vi "Peg-in-hole 2015-03-10 data.vi"() -> ()   [LabVIEW 2013]
uses:
  <vilib>/Analysis/baseanly.llb/Mean (DBL).vi
  <vilib>/Analysis/NI_AALBase.lvlib
  <vilib>/Analysis/NI_AALPro.lvlib
  <vilib>/gmath/NI_Gmath.lvlib
panel:
  in  "Times":dbl[](array[numeric])=[45.5, 55.1, 25.05, 25.0, 25.152, 25.451, 25.3, 25.35, 25.1, 25.25, 14.55, 25.45, 34.85, 25.55, 14.8, 25.15, 86.1, 25.55, 15.2, 25.5, 25.2, 25.201, 15.05, 25.45, 15.0, 25.8, 15.05, 25.1, 15.1, 25.85, 14.9, 25.7, 25.05, 25.1, 46.0, 25.9, 15.3, 25.45, 25.2, 25.601, 14.9, 24.95, 15.2, 25.0, 45.95, 25.25, 385.0, 25.65, 15.3, 25.4, 15.2, 25.7, 14.8, 25.1, 46.75, 25.85, 15.35, 25.1, 15.35, 25.95, 15.6, 25.55, 15.45, 25.45, 14.9, 14.9, 15.1, 15.35, 14.8, 15.05, 56.95, 25.7, 15.0, 15.15, 14.95, 25.899, 15.0, 25.15, 15.4, 15.251, 14.95, 25.6, 15.4, 15.5, 15.15, 14.95, 15.15, 15.25, 15.3, 15.35, 15.251, 15.8, 15.0, 15.05, 15.25, 15.55, 15.55, 15.65, 15.051, 15.5, 15.0, 15.0, 15.1, 15.45, 15.1, 15.15, 15.05, 25.15, 15.15, 15.25, 15.25, 15.1, 14.9, 15.25, 14.85, 15.35, 14.95, 25.85, 15.3, 15.8, 15.2, 15.2, 14.9, 15.3, 14.85, 15.55, 15.25, 15.35, 15.25, 15.3, 14.9, 15.3, 14.85, 15.45, 14.85, 15.3, 15.1, 15.3, 15.05, 15.851]
  in  "y":dbl
  out "correlation coefficient r":dbl
  out "offset":dbl
  out "power":dbl
  out "amplitude":dbl
  out "XY Graph":cluster{cluster{dbl, "mean":dbl}[]}[](graph)
  # "Data using two taught points\n& intervening joint pose"
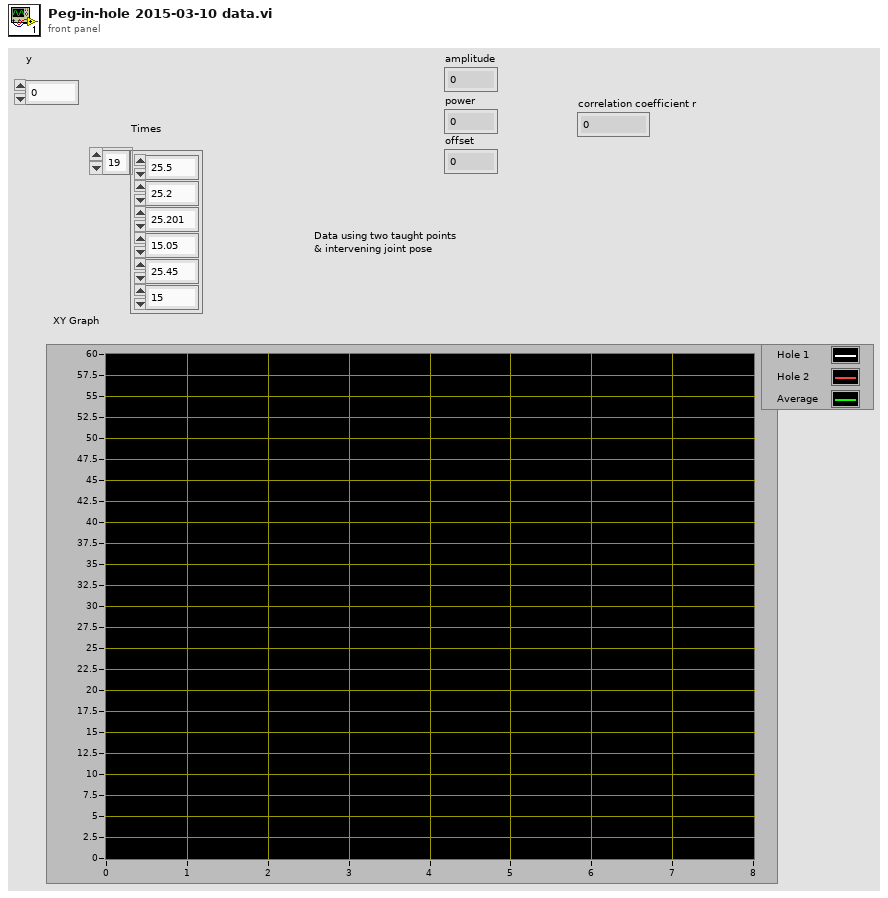
[diagram p1: front panel]
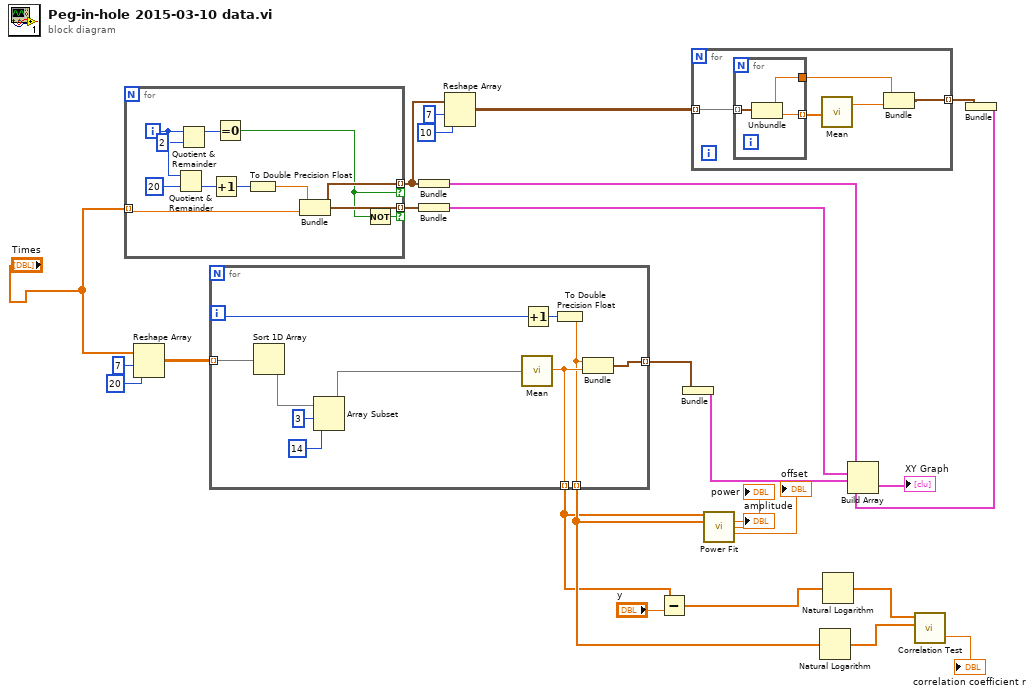
[diagram p0: block diagram]
diagram:
  n1 = for {
    tunnel: "Times" -> [w27] mode=indexing
    tunnel: [w30] -> w22 mode=indexing if=w28
    tunnel: [w30] -> w5 mode=indexing if=w29
    i -> [w33]
    n2 = Quotient & Remainder(x=w33, y=20) -> (floor(x/y)=w36:i32)  [unwired: 1 out]
    n3 = Quotient & Remainder(x=w33, y=2) -> (x-y*floor(x/y)=w31:i32)  [unwired: 1 out]
    n4 = Increment(x=w36) -> (x+1=w35:i32)
    n5 = Equal To 0?(x=w31) -> (x = 0?=w29:bool)
    n6 = To Double Precision Float(number=w35) -> (double precision float=w34:dbl)
    n7 = Bundle(w34, w27) -> (w30:cluster{dbl, dbl})  [unwired: 1 in]
    n8 = Not(x=w29) -> (.not. x?=w28:bool)
  }
  n9 = Reshape Array("Times", 7 ("dimension size"), 20 ("dimension size")) -> (w24:dbl[][])
  n10 = for {
    tunnel: w24 -> [w42] mode=indexing
    tunnel: [w45] -> w23 mode=indexing
    tunnel: [w44] -> w10 mode=indexing
    tunnel: [w43] -> w14 mode=indexing
    i -> [w47]
    n11 = Sort 1D Array(array=w42) -> (sorted array=w39:dbl[])
    n12 = Array Subset(array=w39, index=3, length=14) -> (w38:dbl[])
    n13 = call-poly <vilib>:"Mean.vi"("X"=w38) -> ("mean"=w44:dbl)  [unwired: 1 out]
    n14 = Increment(x=w47) -> (x+1=w46:i32)
    n15 = To Double Precision Float(number=w46) -> (double precision float=w43:dbl)
    n16 = Bundle(w43, "mean"=w44) -> (w45:cluster{dbl, "mean":dbl})  [unwired: 1 in]
  }
  n17 = Bundle(w5) -> (w8:cluster{cluster{dbl, dbl}[]})  [unwired: 1 in]
  n18 = Bundle(w22) -> (w20:cluster{cluster{dbl, dbl}[]})  [unwired: 1 in]
  n19 = Reshape Array(w5, 7 ("dimension size"), 10 ("dimension size")) -> (w4:cluster{dbl, dbl}[][])
  n20 = Subtract(x=w10, y="y") -> (x-y=w9:dbl[])
  n21 = Bundle(w23) -> (w19:cluster{cluster{dbl, "mean":dbl}[]})  [unwired: 1 in]
  n22 = for {
    tunnel: w4 -> [w52] mode=indexing
    tunnel: [w48] -> w3 mode=indexing
    n23 = for {
      tunnel: w52 -> [w55] mode=indexing
      tunnel: [w54] -> w51 mode=indexing
      tunnel: [w53] -> w50
      n24 = Unbundle(w55) -> (w53:dbl, w54:dbl)
    }
    n25 = call-poly <vilib>:"Mean.vi"("X"=w51) -> ("mean"=w49:dbl)  [unwired: 1 out]
    n26 = Bundle(w50, "mean"=w49) -> (w48:cluster{dbl, "mean":dbl})  [unwired: 1 in]
  }
  n27 = call <vilib>:"Power Fit.vi"("Y"=w10, "X"=w14) -> ("amplitude"=→"amplitude":dbl, "power"=→"power":dbl, "offset"=→"offset":dbl)  [unwired: 8 in, 3 out]
  n28 = Natural Logarithm(1:w14) -> (0:w12:dbl[])
  n29 = Natural Logarithm(1:w9) -> (0:w13:dbl[])
  n30 = call <vilib>:"Correlation Test.vi"("sample set y"=w12, "sample set x"=w13) -> ("correlation coefficient r"=→"correlation coefficient r":dbl)  [unwired: 5 in, 4 out]
  n31 = Bundle(w3) -> (w2:cluster{cluster{dbl, "mean":dbl}[]})  [unwired: 1 in]
  n32 = Build Array(w8, w20, w19, w2) -> (→"XY Graph":cluster{cluster{dbl, "mean":dbl}[]}[])
